vi "Do.vi"(8 "error in (no error)":errorcluster, 10 "Actor in":refnum<class "Actor.lvclass">, 11 "Close Msg":refnum<class "Close Msg.lvclass">) -> (0 "error out":errorcluster, 2 "Actor out":refnum<class "Actor.lvclass">)   [LabVIEW 2016, in "Function Actor.lvlib" / "Close Msg.lvclass"]
uses:
  <userlib>/Common Components/Function Actor/Messages/Close Msg/Close Msg.lvclass
  <vilib>/ActorFramework/Actor/Actor.lvclass
  <userlib>/Common Components/Function Actor/Function.lvclass
  C:/Program Files (x86)/National Instruments/LabVIEW 2016/vi.lib/ActorFramework/Actor/Actor.lvclass
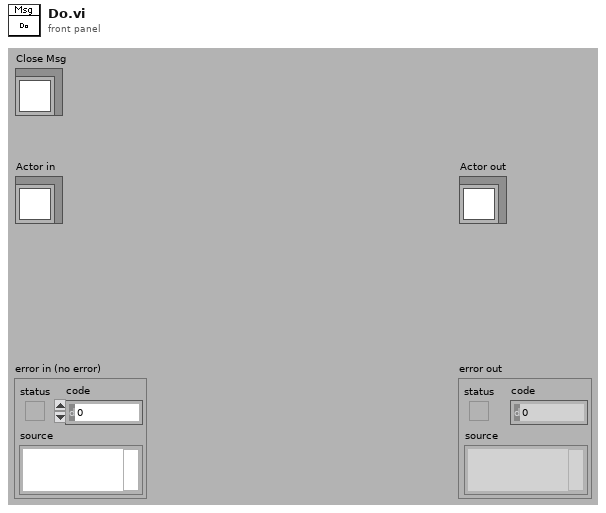
[diagram p1: front panel]
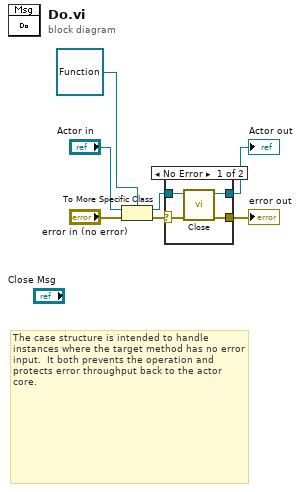
[diagram p0: block diagram]
diagram:
  # "The case structure is intended to handle instances where the target method has no error input.  It both prevents the operation and protects error throughput back to the actor core."
  n1 = To More Specific Class(target class=refnum<class "Function.lvclass"> refnum ("Actor in"), reference="Actor in", error in="error in (no error)") -> (specific class reference=w7:refnum<class "Function.lvclass">, error out=w3:errorcluster)
  n2 = case shown="No Error" w3 {
    selector: w3 -> [w8 w13]
    tunnel: w7 -> [w11 w12]
    tunnel: [w10 w13] -> w2
    tunnel: [w9 w12] -> w1
    frame No Error {
      n3 = call-dynamic "Close.vi"("error in (no error)"=w8, "Function in"=w11) -> ("error out"=w10:errorcluster, "Function out"=w9:refnum<class "Function.lvclass">)  [unwired: 8 in]
    }
    frame Error {
    }
  }
  "error out" <- w2
  "Actor out" <- w1
